vi "Disable Controls.vi"(5 "Disabled State":u8, 7 "Control Names":string[](array[string]), 9 "Control Refs":refnum<vi>[](array[refnum])) -> ()   [LabVIEW 2011]
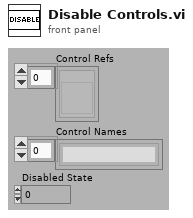
[diagram p1: front panel]
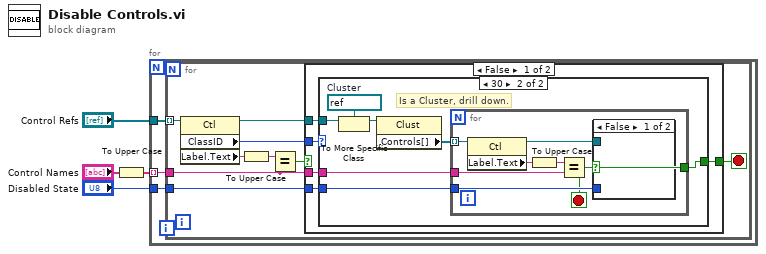
[diagram p0: block diagram]
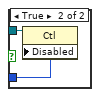
[diagram p3: hidden frame]
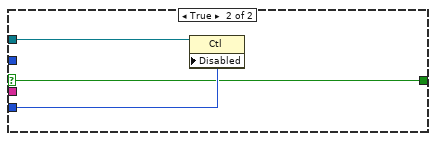
[diagram p4: hidden frame]
diagram:
  n1 = To Upper Case(1:"Control Names") -> (0:w1:string[])
  n2 = for {
    tunnel: "Control Refs" -> [w7]
    tunnel: w1 -> [w6] mode=indexing
    tunnel: "Disabled State" -> [w5]
    n3 = for {
      tunnel: w7 -> [w16] mode=indexing
      tunnel: w6 -> [w10]
      tunnel: w5 -> [w12]
      stop <- w11 stop-if-true
      n4 = property class="Ctl"(reference=w16) -> (reference out=w14:refnum<vi>, "ClassID"=w13:u32, "Label.Text"=w9:string)  [unwired: 1 in, 1 out]
      n5 = To Upper Case(1:w9) -> (0:w8:string)
      n6 = Equal?(x=w8, y=w10) -> (x = y?=w15:bool)
      n7 = case shown="False" w15 {
        selector: w15 -> [_ w38]
        tunnel: w14 -> [w20 w40]
        tunnel: w13 -> [w21 _]
        tunnel: w12 -> [w18 w39]
        tunnel: [w17 w38] -> w11
        tunnel: w10 -> [w19 _]
        frame False {
          n8 = case shown="30" w21 {
            tunnel: w20 -> [_ w28]
            tunnel: w19 -> [_ w24]
            tunnel: w18 -> [_ w23]
            tunnel: [_ w22] -> w17
            frame Default {
            }
            frame 30 {
              w27 = refnum<vi> refnum  # Cluster
              # "Is a Cluster, drill down."
              n9 = To More Specific Class(target class=w27, reference=w28) -> (specific class reference=w26:refnum<vi>)  [unwired: 1 in, 1 out]
              n10 = property class="Clust"(reference=w26) -> ("Controls[]"=w25:refnum<vi>[])  [unwired: 1 in, 2 out]
              n11 = for {
                tunnel: w25 -> [w35] mode=indexing
                tunnel: w24 -> [w33]
                tunnel: w23 -> [w30]
                tunnel: [w29] -> w22
                stop <- w29 stop-if-true
                n12 = property class="Ctl"(reference=w35) -> (reference out=w31:refnum<vi>, "Label.Text"=w34:string)  [unwired: 1 in, 1 out]
                n13 = To Upper Case(1:w34) -> (0:w32:string)
                n14 = Equal?(x=w32, y=w33) -> (x = y?=w29:bool)
                n15 = case shown="False" w29 {
                  tunnel: w31 -> [_ w37]
                  tunnel: w30 -> [_ w36]
                  frame False {
                  }
                  frame True {
                    n16 = property class="Ctl"(reference=w37, "Disabled"=w36) -> ()  [unwired: 1 in, 2 out]
                  }
                }
              }
            }
          }
        }
        frame True {
          n17 = property class="Ctl"(reference=w40, "Disabled"=w39) -> ()  [unwired: 1 in, 2 out]
        }
      }
    }
  }
